vi "Autonomous Independent.vi"() -> ()   [LabVIEW 2016]
doc: "This VI is called when autonomous begins, and will automatically be terminated when autonomous ends. You can carry out timed or sensor driven robot movement independently without needing to return to the caller."
uses:
  <vilib>/Rock Robotics/WPI/ThirdParty/CanMotor/TalonSRX/WPI_CANTalonSRX_APIControlMode.ctl
  <vilib>/Rock Robotics/WPI/ThirdParty/CanMotor/TalonSRX/WPI_CANTalonSRX_APIFeedbackSelect.ctl
  <vilib>/Rock Robotics/WPI/Solenoid/WPI_SolenoidValue.ctl
  <vilib>/Rock Robotics/WPI/Utilities/WPI_GetSetVariantRefNum.vi
  <vilib>/Rock Robotics/Network Tables/NT Read String.vi
  <vilib>/Rock Robotics/WPI/Solenoid/WPI_SolenoidSetEnum.vi
  <vilib>/Rock Robotics/Network Tables/NT Write Numeric Array.vi
panel:
  in  "Output":dbl format="%#_13g"
  in  "Target Position":dbl format="%#_13g"
  in  "F":dbl
  in  "D":dbl
  in  "I":dbl
  in  "P":dbl
  # "Percent output for the motors pull away from the tower"
  # "Be sure to right-click and choose Data Operations>>Make Current Value default if you want to save the array values with the VI"
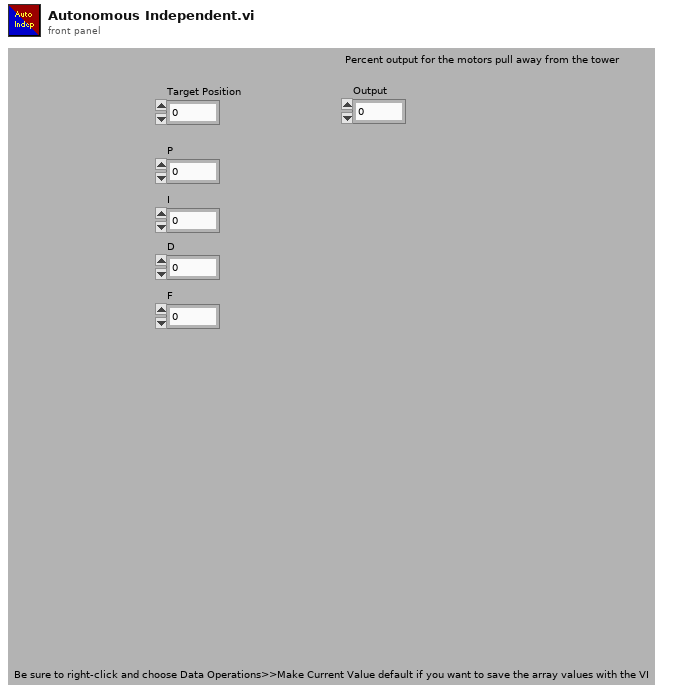
[diagram p1: front panel]
types:
  T1 = typedef "WPI_JoystickDevRef.ctl" = cluster{"Device":T2}
  T2 = typedef "WPI_JoystickDeviceEnum.ctl" = enum16{"USB 0", "USB 1", "USB 2", "USB 3", "USB 4", "USB 5"}
  T3 = typedef "WPI_CANTalonSRX_APIControlMode.ctl" = enum8{"Percent VBus", "Speed", "Position", "Slave", "Unchanged / Invalid", "Voltage Compensation", "Current", "Motion Profile", "Motion Magic"}
  T4 = typedef "WPI_SolenoidValue.ctl" = enum16{"Off", "On", "Forward", "Reverse"}
  T5 = typedef "WPI_MotorControlDeviceRef.ctl" = cluster{"DeviceStatus":errorcluster, "Type":T6, "PWM":cluster{"PWM Channel":T7, "DeadBand":T8}, "CAN":cluster{"Device Number":u8, "SetOutput VI Ref":variant, "GetOutput VI Ref":variant, "Enable VI Ref":variant, "Disable VI Ref":variant, "Data":variant}, "Invert":bool}
  T6 = typedef "WPI_MotorControlType.ctl" = enum16{"PWM", "CAN"}
  T7 = typedef "FPGA_DIOPWMChannel.ctl" = enum8{"PWM 0", "PWM 1", "PWM 2", "PWM 3", "PWM 4", "PWM 5", "PWM 6", "PWM 7", "PWM 8", "PWM 9", "PWM MXP 0", "PWM MXP 1", "PWM MXP 2", "PWM MXP 3", "PWM MXP 4", "PWM MXP 5", "PWM MXP 6", "PWM MXP 7", "PWM MXP 8", "PWM MXP 9", "Invalid"}
  T8 = typedef "WPI_PWMDeadband.ctl" = cluster{"Name":string, "maxPositivePwm":i32, "minPositivePwm":i32, "centerPwm":i32, "maxNegativePwm":i32, "minNegativePwm":i32, "angularRange":u16}
  T9 = typedef "WPI_CANTalonSRX_APIFeedbackSelect.ctl" = enum16{"Digital Quadrature Encoder", "Analog Potentiometer", "Analog Encoder", "Count on Quad-A (Rising-Edge)", "Count on Quad-A (Falling-Edge)", "CTR Magnetic Enc (Absolute)", "CTR Magnetic Enc (Relative)", "Pulse Width"}
  T10 = typedef "WPI_SolenoidDevRef.ctl" = cluster{"DevStatus":errorcluster, "Pneumatics Control Module":u8, "Forward Solenoid Channel":T11, "Reverse Solenoid Channel":T11}
  T11 = typedef "WPI_SolenoidChannel.ctl" = enum8{"Solenoid 0", "Solenoid 1", "Solenoid 2", "Solenoid 3", "Solenoid 4", "Solenoid 5", "Solenoid 6", "Solenoid 7", "Invalid"}
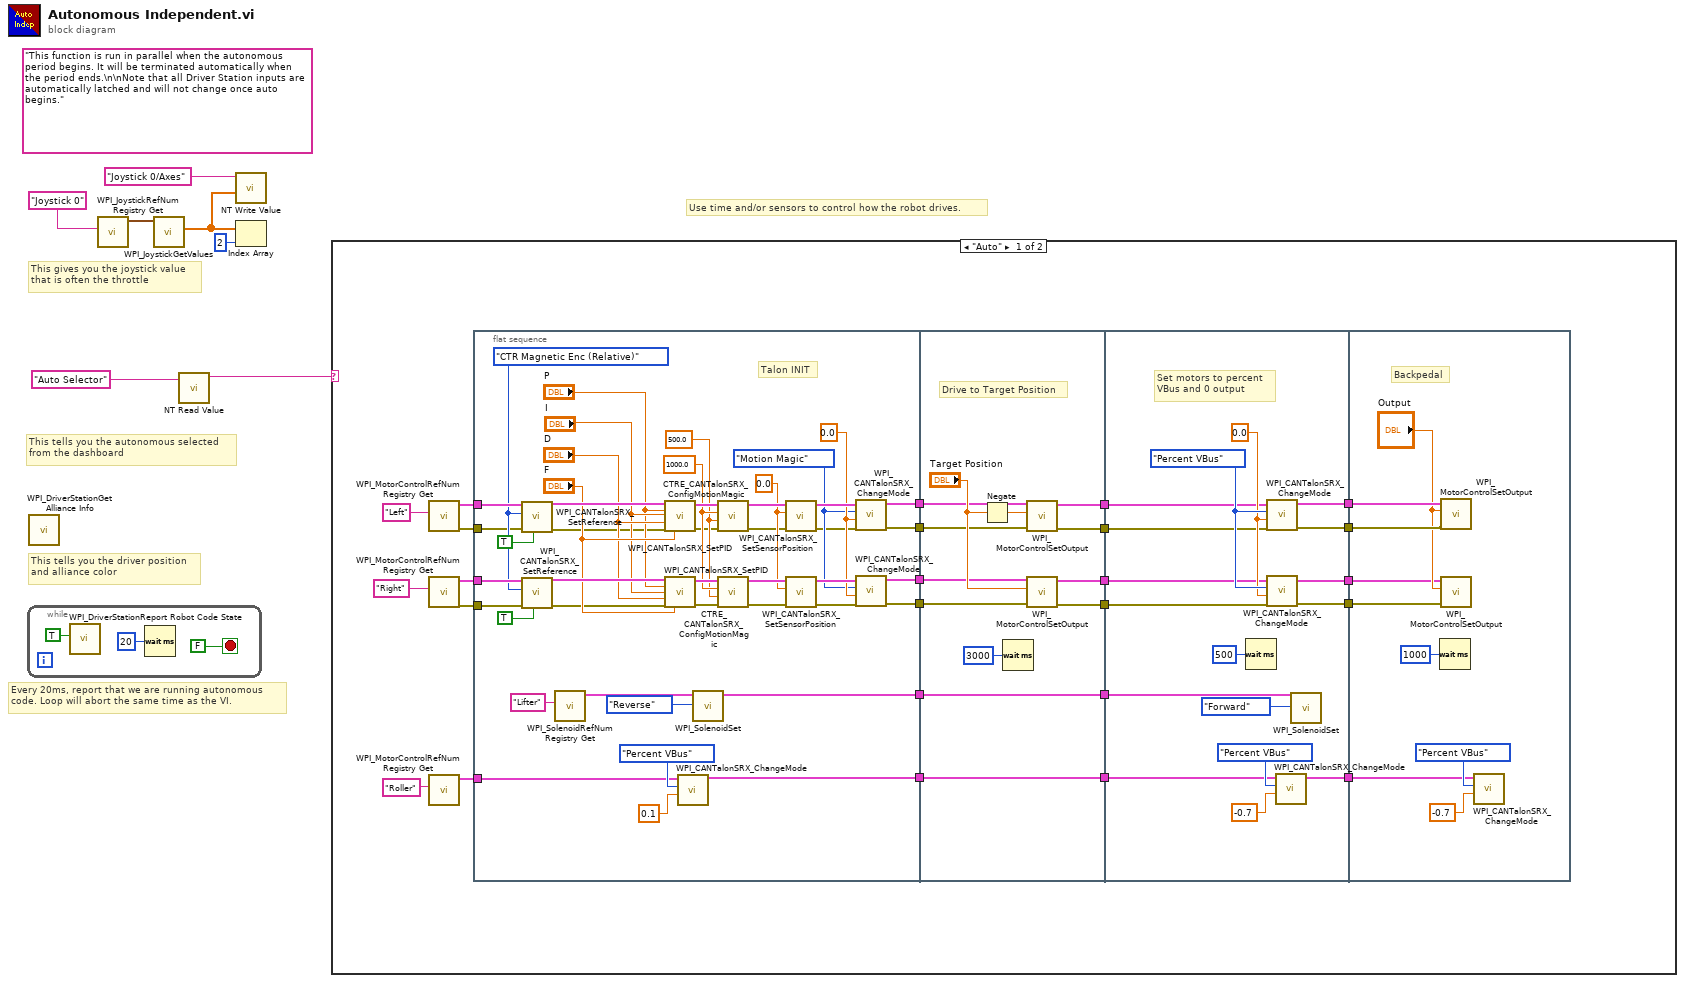
[diagram p0: block diagram]
diagram:
  (unwired) "This function is run in parallel when the autonomous period begins. It will be terminated automatically when the period ends.\n\nNote that all Driver Station inputs are automatically latched and will not change once auto begins."
  # "This tells you the autonomous selected\nfrom the dashboard"
  # "Every 20ms, report that we are running autonomous\ncode. Loop will abort the same time as the VI."
  # "This gives you the joystick value\nthat is often the throttle"
  # "Use time and/or sensors to control how the robot drives."
  # "This tells you the driver position\nand alliance color"
  n1 = while {
    stop <- FALSE stop-if-true
    n2 = call <vilib>:"WPI_DriverStationReport Robot Code State.vi"("Autonomous"=TRUE) -> ()  [unwired: 10 in, 1 out]
    n3 = Wait (ms)(milliseconds to wait=u32 20) -> ()  [unwired: 1 out]
  }
  n4 = call <vilib>:"WPI_DriverStationGet Alliance Info.vi"() -> ()  [unwired: 12 out]
  n5 = call <vilib>:"WPI_JoystickRefNum Registry Get.vi"("refnum name"="Joystick 0") -> ("JoystickDevRef"=w6:T1)  [unwired: 1 in, 9 out]
  n6 = call <vilib>:"WPI_JoystickGetValues.vi"("JoystickDevRef"=w6) -> ("Axes"=w2:dbl[])  [unwired: 6 in, 4 out]
  n7 = call-poly <vilib>:"NT Read Value.vi"("Name"="Auto Selector") -> ("String"=w3:string)  [unwired: 9 in, 1 out]
  n8 = call-poly <vilib>:"NT Write Value.vi"("Numeric Array"=w2, "Name"="Joystick 0/Axes") -> ()  [unwired: 9 in, 1 out]
  n9 = Index Array(array=w2, index=2) -> ()  [unwired: 1 out]
  n10 = case shown="\"Auto\"" w3 {
    frame "Auto" {
      n11 = call <vilib>:"WPI_MotorControlRefNum Registry Get.vi"("refnum name"="Left") -> ("error out"=w31:errorcluster, "MotorControlDevRef"=w35:T5)  [unwired: 9 in]
      n12 = call <vilib>:"WPI_MotorControlRefNum Registry Get.vi"("refnum name"="Right") -> ("error out"=w30:errorcluster, "MotorControlDevRef"=w34:T5)  [unwired: 9 in]
      n13 = call <vilib>:"WPI_MotorControlRefNum Registry Get.vi"("refnum name"="Roller") -> ("MotorControlDevRef"=w16:T5)  [unwired: 9 in, 1 out]
      n14 = flat-sequence {
        tunnel: w35 -> [w75]
        tunnel: w34 -> [w70]
        tunnel: w31 -> [w59]
        tunnel: w30 -> [w54]
        tunnel: [w49] -> w29
        tunnel: [w48] -> w28
        tunnel: [w47] -> w27
        tunnel: [w46] -> w26
        tunnel: w16 -> [w40]
        tunnel: [w39] -> w15
        tunnel: [w38] -> w12
        tunnel: w29 -> [w91]
        tunnel: w28 -> [w90]
        tunnel: w27 -> [w89]
        tunnel: w26 -> [w88]
        tunnel: [w86] -> w25
        tunnel: [w85] -> w24
        tunnel: [w84] -> w23
        tunnel: [w83] -> w22
        tunnel: w15 -> [w82]
        tunnel: [w82] -> w14
        tunnel: [w81] -> w13
        tunnel: w12 -> [w81]
        tunnel: w25 -> [w107]
        tunnel: w24 -> [w106]
        tunnel: w23 -> [w105]
        tunnel: w22 -> [w104]
        tunnel: [w103] -> w21
        tunnel: [w102] -> w20
        tunnel: [w101] -> w19
        tunnel: [w100] -> w18
        tunnel: w14 -> [w95]
        tunnel: w13 -> [w94]
        tunnel: [w93] -> w11
        tunnel: w21 -> [w118]
        tunnel: w20 -> [w117]
        tunnel: w19 -> [w115]
        tunnel: w18 -> [w114]
        tunnel: w11 -> [w110]
        frame #0 {
          w67 = 500.0 ("Max Acceleration")
          w68 = 1000.0 ("Cruise Velocity")
          w69 = WPI_CANTalonSRX_APIFeedbackSelect."CTR Magnetic Enc (Relative)" ("Feedback Reference")
          w65 = 0.0 ("Output")
          w66 = 0.0 ("New Sensor Position")
          w64 = WPI_CANTalonSRX_APIControlMode."Motion Magic" ("Control Mode")
          # "Talon INIT"
          n15 = call <vilib>:"WPI_CANTalonSRX_SetReference.vi"("Reverse Closed-Loop Output"=TRUE, "error in (no error)"=w59, "Feedback Reference"=w69, "CAN Talon SRX Ref"=w75) -> ("error out"=w58:errorcluster, "CAN Talon SRX Ref"=w78:T5)  [unwired: 6 in]
          n16 = call <vilib>:"WPI_CANTalonSRX_SetReference.vi"("Reverse Closed-Loop Output"=TRUE, "error in (no error)"=w54, "Feedback Reference"=w69, "CAN Talon SRX Ref"=w70) -> ("error out"=w53:errorcluster, "CAN Talon SRX Ref"=w72:T5)  [unwired: 6 in]
          n17 = call <vilib>:"WPI_SolenoidRefNum Registry Get.vi"("refnum name"="Lifter") -> ("SolenoidDevRef"=w43:T10)  [unwired: 9 in, 1 out]
          n18 = call <vilib>:"WPI_CANTalonSRX_SetPID.vi"("CAN Talon SRX Ref"=w78, "P"="P", "I"="I", "D"="D", "error in (no error)"=w58, "F"="F") -> ("CAN Talon SRX Ref"=w79:T5, "error out"=w57:errorcluster)  [unwired: 8 in]
          n19 = call <vilib>:"WPI_CANTalonSRX_SetPID.vi"("CAN Talon SRX Ref"=w72, "P"="P", "I"="I", "D"="D", "error in (no error)"=w53, "F"="F") -> ("CAN Talon SRX Ref"=w71:T5, "error out"=w52:errorcluster)  [unwired: 8 in]
          n20 = call <vilib>:"WPI_CANTalonSRX_ChangeMode.vi"("Output"=0.1 ("Roll Out Output"), "Control Mode"=WPI_CANTalonSRX_APIControlMode."Percent VBus", "CAN Talon SRX Ref"=w40) -> ("CAN Talon SRX Ref"=w39:T5)  [unwired: 7 in, 1 out]
          n21 = call-poly <vilib>:"WPI_SolenoidSet.vi"("Value"=WPI_SolenoidValue."Reverse", "SolenoidDevRef"=w43) -> ("SolenoidDevRef"=w38:T10)  [unwired: 8 in, 1 out]
          n22 = call <vilib>:"CTRE_CANTalonSRX_ConfigMotionMagic.vi"("error in (no error)"=w57, "Max Acceleration"=w67, "Cruise Velocity"=w68, "CAN Talon SRX Ref"=w79) -> ("error out"=w56:errorcluster, "CAN Talon SRX Ref Out"=w77:T5)  [unwired: 6 in]
          n23 = call <vilib>:"CTRE_CANTalonSRX_ConfigMotionMagic.vi"("error in (no error)"=w52, "Max Acceleration"=w67, "Cruise Velocity"=w68, "CAN Talon SRX Ref"=w71) -> ("error out"=w51:errorcluster, "CAN Talon SRX Ref Out"=w73:T5)  [unwired: 6 in]
          n24 = call <vilib>:"WPI_CANTalonSRX_SetSensorPosition.vi"("error in (no error)"=w56, "New Sensor Position"=w66, "CAN Talon SRX Ref"=w77) -> ("error out"=w55:errorcluster, "CAN Talon SRX Ref"=w76:T5)  [unwired: 7 in]
          n25 = call <vilib>:"WPI_CANTalonSRX_SetSensorPosition.vi"("error in (no error)"=w51, "New Sensor Position"=w66, "CAN Talon SRX Ref"=w73) -> ("error out"=w50:errorcluster, "CAN Talon SRX Ref"=w74:T5)  [unwired: 7 in]
          n26 = call <vilib>:"WPI_CANTalonSRX_ChangeMode.vi"("error in (no error)"=w55, "Output"=w65, "Control Mode"=w64, "CAN Talon SRX Ref"=w76) -> ("error out"=w48:errorcluster, "CAN Talon SRX Ref"=w49:T5)  [unwired: 6 in]
          n27 = call <vilib>:"WPI_CANTalonSRX_ChangeMode.vi"("error in (no error)"=w50, "Output"=w65, "Control Mode"=w64, "CAN Talon SRX Ref"=w74) -> ("error out"=w46:errorcluster, "CAN Talon SRX Ref"=w47:T5)  [unwired: 6 in]
        }
        frame #1 {
          # "Drive to Target Position"
          n28 = Negate(x="Target Position") -> (-x=w80:dbl)
          n29 = Wait (ms)(milliseconds to wait=u32 3000) -> ()  [unwired: 1 out]
          n30 = call <vilib>:"WPI_MotorControlSetOutput.vi"("error in (no error)"=w90, "Output"=w80, "MotorControlDevRef"=w91) -> ("error out"=w85:errorcluster, "MotorControlDevRef"=w86:T5)  [unwired: 6 in, 1 out]
          n31 = call <vilib>:"WPI_MotorControlSetOutput.vi"("error in (no error)"=w88, "Output"="Target Position", "MotorControlDevRef"=w89) -> ("error out"=w84:errorcluster, "MotorControlDevRef"=w83:T5)  [unwired: 6 in, 1 out]
        }
        frame #2 {
          w108 = 0.0 ("Output")
          w109 = WPI_CANTalonSRX_APIControlMode."Percent VBus" ("Control Mode")
          # "Set motors to percent \nVBus and 0 output"
          n32 = Wait (ms)(milliseconds to wait=u32 500) -> ()  [unwired: 1 out]
          n33 = call <vilib>:"WPI_CANTalonSRX_ChangeMode.vi"("error in (no error)"=w106, "Output"=w108, "Control Mode"=w109, "CAN Talon SRX Ref"=w107) -> ("error out"=w102:errorcluster, "CAN Talon SRX Ref"=w103:T5)  [unwired: 6 in]
          n34 = call <vilib>:"WPI_CANTalonSRX_ChangeMode.vi"("error in (no error)"=w105, "Output"=w108, "Control Mode"=w109, "CAN Talon SRX Ref"=w104) -> ("error out"=w100:errorcluster, "CAN Talon SRX Ref"=w101:T5)  [unwired: 6 in]
          n35 = call <vilib>:"WPI_CANTalonSRX_ChangeMode.vi"("Output"=-0.7 ("Roll Out Output"), "Control Mode"=WPI_CANTalonSRX_APIControlMode."Percent VBus", "CAN Talon SRX Ref"=w95) -> ("CAN Talon SRX Ref"=w93:T5)  [unwired: 7 in, 1 out]
          n36 = call-poly <vilib>:"WPI_SolenoidSet.vi"("Value"=WPI_SolenoidValue."Forward", "SolenoidDevRef"=w94) -> ()  [unwired: 8 in, 2 out]
        }
        frame #3 {
          # "Backpedal"
          n37 = Wait (ms)(milliseconds to wait=u32 1000) -> ()  [unwired: 1 out]
          n38 = call <vilib>:"WPI_MotorControlSetOutput.vi"("error in (no error)"=w117, "Output"="Output", "MotorControlDevRef"=w118) -> ()  [unwired: 6 in, 3 out]
          n39 = call <vilib>:"WPI_MotorControlSetOutput.vi"("error in (no error)"=w114, "Output"="Output", "MotorControlDevRef"=w115) -> ()  [unwired: 6 in, 3 out]
          n40 = call <vilib>:"WPI_CANTalonSRX_ChangeMode.vi"("Output"=-0.7 ("Roll Out Output"), "Control Mode"=WPI_CANTalonSRX_APIControlMode."Percent VBus", "CAN Talon SRX Ref"=w110) -> ()  [unwired: 7 in, 2 out]
        }
      }
    }
    frame Default {
      # "You can put your main auto here, or you can right-click on the case and make any\nother frame be the default case."
      # "This is the frame that will execute if no selection is made, or if it is not recognized"
    }
  }
